vi "Compute DistanceTo Coral2.vi"(6 "Robot Calibration Cluster":T2={"Camera Height on robot (in)"=34.5, "Camera Angle on the robot (deg)"=28.3, "Camera FOV Top to Bottom View Angle (deg)"=0.946, "Target size (in)"=6.5, "Distance to front of bumper (in)"=9.75, "Focal Length (mm)"=10.0, "Yaw Slope"=1.0} {"Focal Length (mm)" format="%#_13g"; "Distance to front of bumper (in)" format="%#_13g"; "Target size (in)" format="%#_13g"; "Camera FOV Top to Bottom View Angle (deg)" format="%#_13g"; "Camera Angle on the robot (deg)" format="%#_13g"; "Camera Height on robot (in)" format="%#_13g"}, 8 "results 2":T1, 10 "FOV Left to Right (deg)":dbl=68.5 format="%#_13g", 11 "Image Src":T3) -> (0 "results out":T1, 2 "Offset Angle":dbl=569.258018632146, 3 "Image Dst Out":T3, 4 "Distance from target (in)":dbl=116.40675998176638 format="%.2f")   [LabVIEW 2023]
doc: "Using the camera lens information and the real world size of the target, use trig and ratios to determine the distance to the target. Also returns the location relative to the image center in a (-1 , 1) coordinate system that may be useful for steering the robot."
uses:
  <vilib>/vision/Image Controls.llb/IMAQ Image.ctl
  April Tags/Camera Info.ctl
  Target Fields.ctl
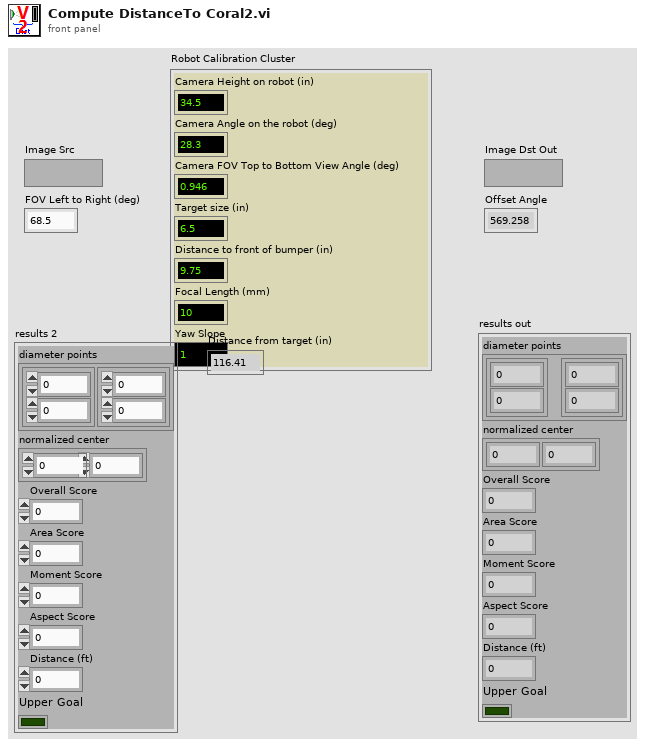
[diagram p1: front panel]
types:
  T1 = typedef "Target Fields.ctl" = cluster{"diameter points":cluster{"first point":cluster{"x":dbl, "y":dbl}, "projected point":cluster{"x":dbl, "y":dbl}}, "normalized center":cluster{"x":dbl, "y":dbl}, "Overall Score":dbl, "Area Score":dbl, "Moment Score":dbl, "Aspect Score":dbl, "Distance (ft)":dbl, "Upper Goal":bool}
  T2 = typedef "Camera Info.ctl" = cluster{"Camera Height on robot (in)":dbl, "Camera Angle on the robot (deg)":dbl, "Camera FOV Top to Bottom View Angle (deg)":dbl, "Target size (in)":dbl, "Distance to front of bumper (in)":dbl, "Focal Length (mm)":dbl, "Yaw Slope":dbl}
  T3 = typedef "IMAQ Image.ctl" = refnum<image>
  T4 = cluster{"first point":cluster{"x":dbl, "y":dbl}, "projected point":cluster{"x":dbl, "y":dbl}}
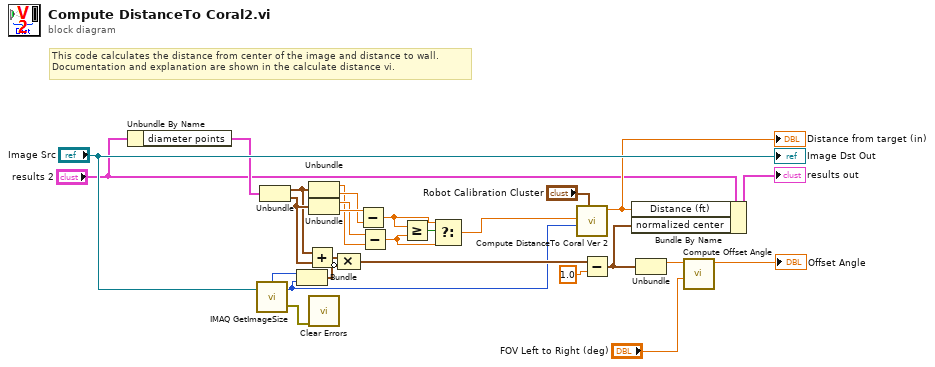
[diagram p0: block diagram]
diagram:
  # "This code calculates the distance from center of the image and distance to wall.\nDocumentation and explanation are shown in the calculate distance vi."
  n1 = Unbundle By Name("results 2") -> ("diameter points"=w9:T4)
  n2 = call "IMAQ GetImageSize"("Image"="Image Src") -> ("Y Resolution"=w17:i32, "X Resolution"=w18:i32, "error out"=w27:errorcluster)  [unwired: 3 in]
  n3 = Unbundle(w9) -> ("first point"=w13:cluster{"x":dbl, "y":dbl}, "projected point"=w16:cluster{"x":dbl, "y":dbl})
  n4 = Bundle("X Resolution"=w18, "Y Resolution"=w17) -> (w12:cluster{"X Resolution":i32, "Y Resolution":i32})  [unwired: 1 in]
  n5 = Add(x=w13, y=w16) -> (x+y=w24:cluster{"x":dbl, "y":dbl})
  n6 = Unbundle(w13) -> ("x"=w1:dbl, "y"=w14:dbl)
  n7 = Unbundle(w16) -> ("x"=w2:dbl, "y"=w15:dbl)
  n8 = call <vilib>:"Clear Errors.vi"("error in (no error)"=w27) -> ()  [unwired: 5 in, 2 out]
  n9 = Compound Arithmetic op=MULTIPLY(w24, invert w12) -> (w25:cluster{dbl, dbl})
  n10 = Subtract(x=w15, y=w14) -> (x-y=w5:dbl)
  n11 = Subtract(x=w2, y=w1) -> (x-y=w4:dbl)
  n12 = Greater Or Equal?(x=w5, y=w4) -> (x >= y?=w6:bool)
  n13 = Select(t=w5, s=w6, f=w4) -> (s? t:f=w3:dbl)
  n14 = call "Compute DistanceTo Coral Ver 2.vi"("Robot Calibration Cluster"="Robot Calibration Cluster", "Screen resolution pixels Height (Ry)"=w17, "Target Vertical pixels bottom - top (pixels)"=w3) -> ("Distance from target (in)"=w10:dbl)  [unwired: 8 in]
  "Distance from target (in)" <- w10
  n15 = Subtract(x=w25, y=1.0) -> (x-y=w21:cluster{dbl, dbl})
  n16 = Bundle By Name(cluster="results 2", "Distance (ft)"=w10, "normalized center"=w21) -> (→"results out":T1)
  n17 = Unbundle(w21) -> (w20:dbl)  [unwired: 1 out]
  n18 = call "Compute Offset Angle.vi"("Field of view"="FOV Left to Right (deg)", "Offset Normilized"=w20) -> ("Offset Angle"=→"Offset Angle":dbl)  [unwired: 9 in]
  "Image Dst Out" <- "Image Src"
